vi "Motor Control (State Machine).vi"() -> ()   [LabVIEW 2013]
uses:
  <vilib>/eio/EIONode/EIONode.xnode
  <vilib>/rvi/eio/common/nirviEmuTemplateMethod_errors.vi
panel:
  in  "stop":bool
  in  "Update":bool
  out "Inside values":T1
  in  "Control":T1={"Pulse Lenght DIO3"=10000, "Pulse Period 3"=20000, "Angle"=0}
  in  "Position Reset":bool
  out "Position (Counts)":i64
  in  "Velocity Interval (uSec)":u64
  out "Acceleration (Counts/Interval)":i64
  out "Velocity (Counts/Interval)":i64
  out "Tours":i64
  out "Degree (relative)":i64
  out "Degree (absolute)":i64
  out "Pulses":i64
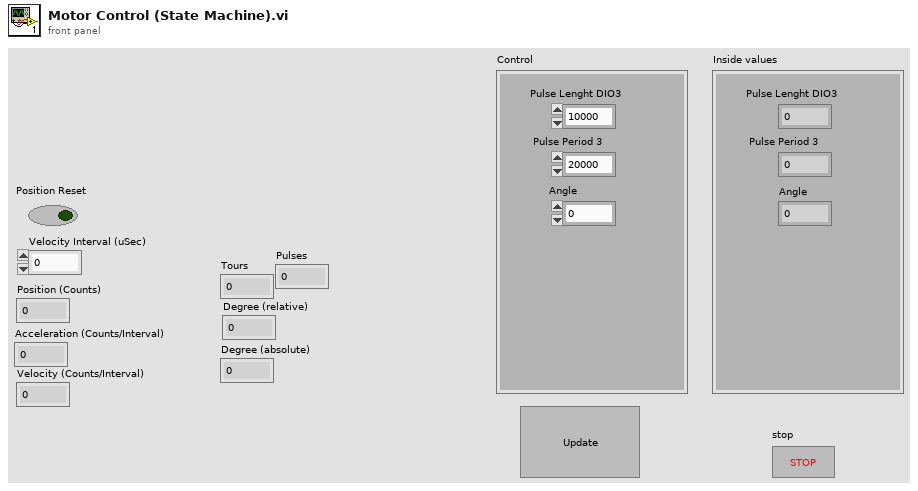
[diagram p1: front panel]
types:
  T1 = cluster{"Pulse Lenght DIO3":i16, "Pulse Period 3":i16, "Angle":i16}
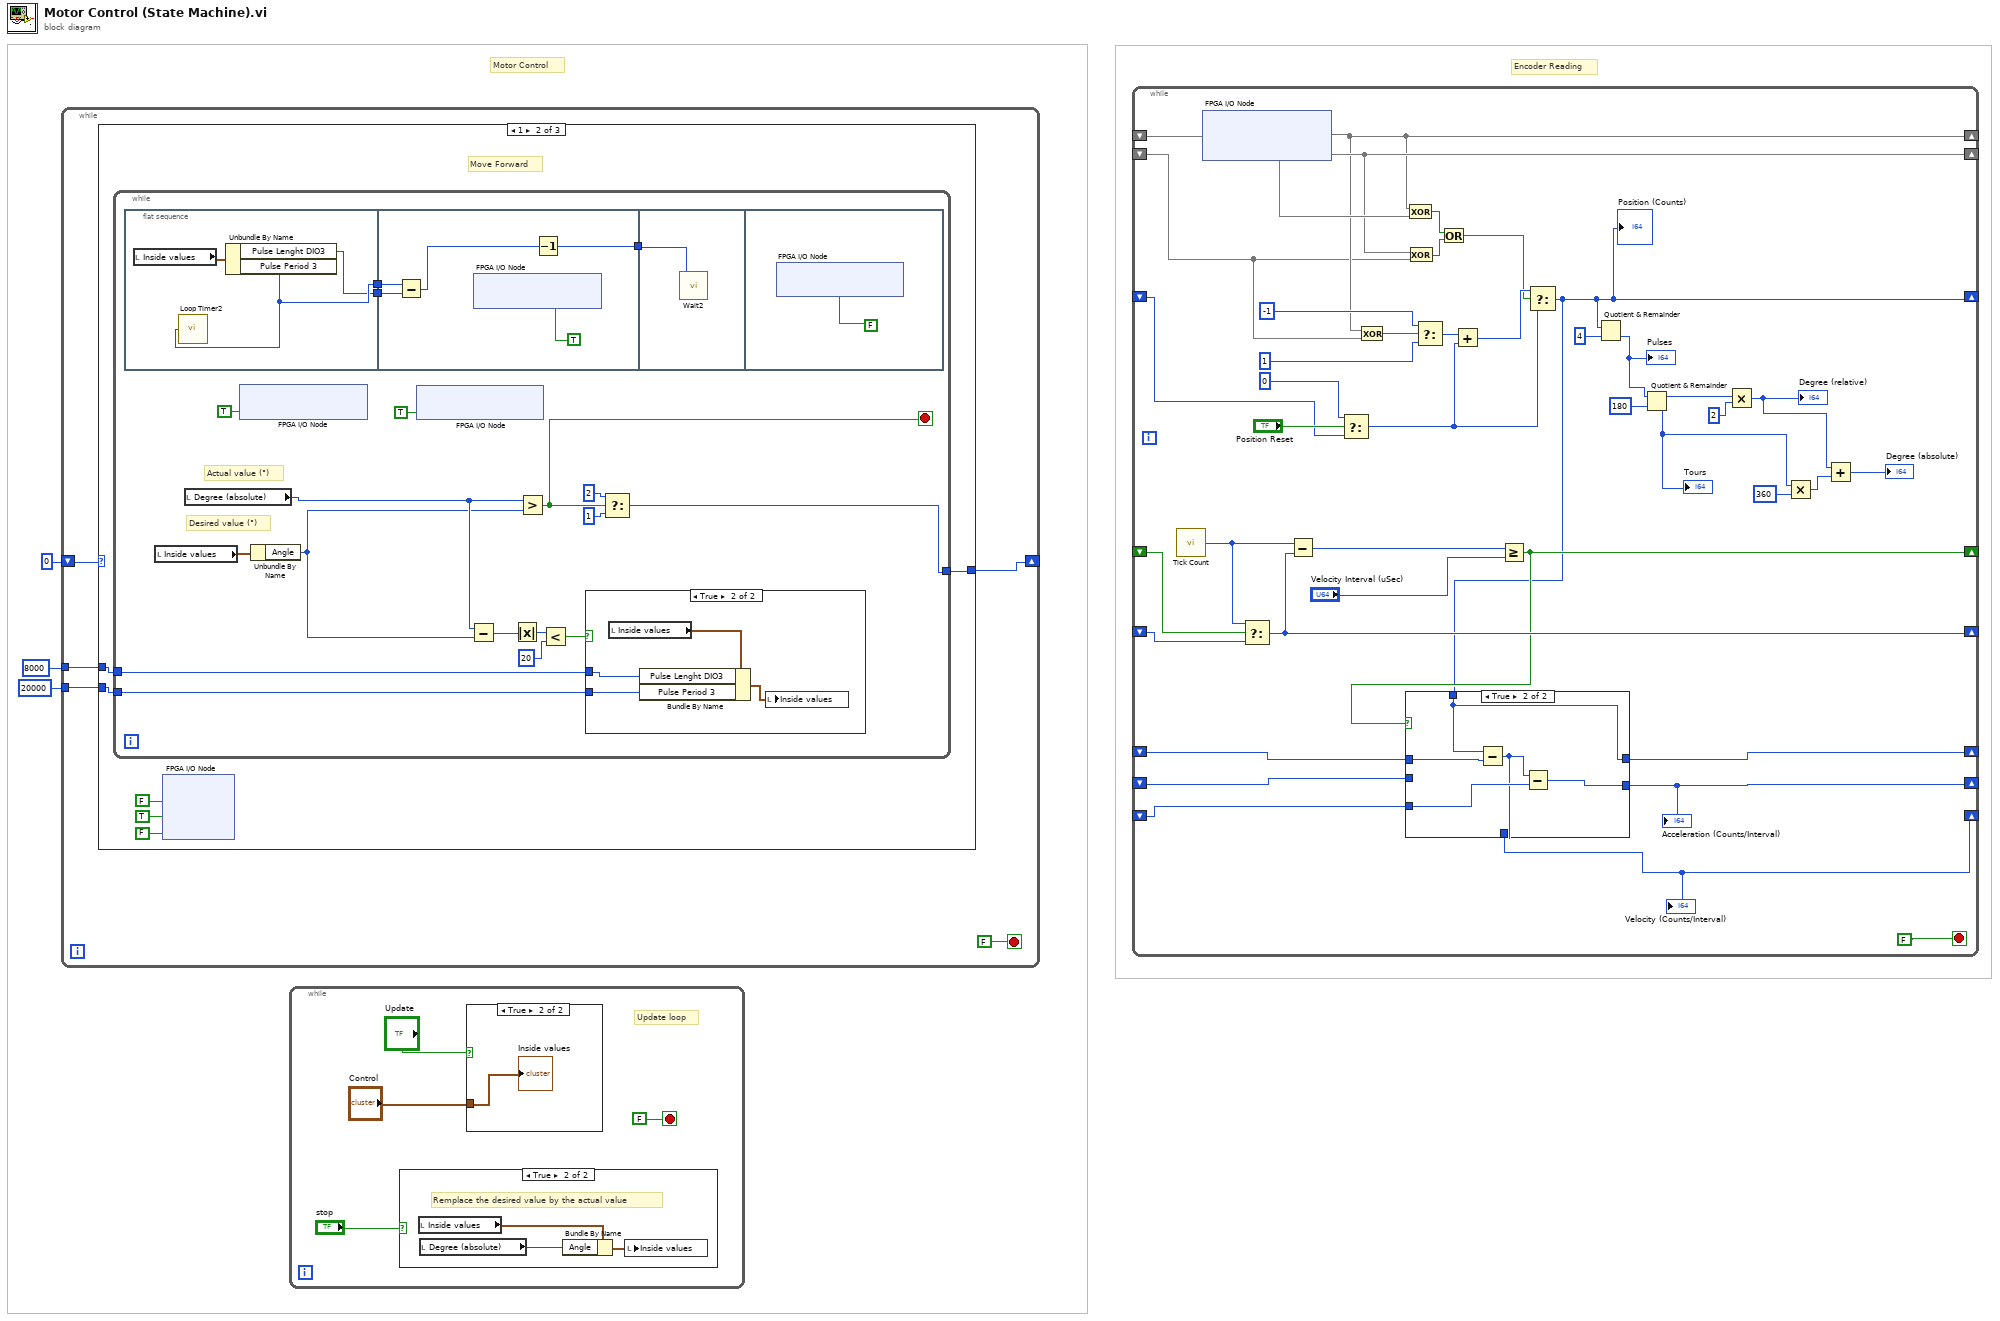
[diagram p0: block diagram]
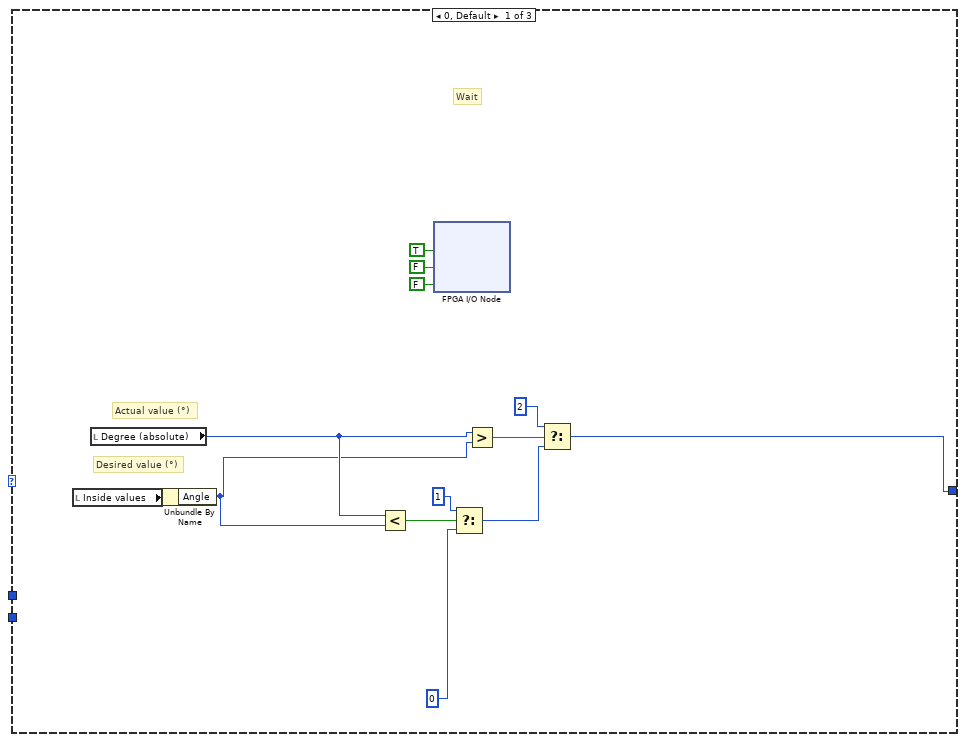
[diagram p5: hidden frame]
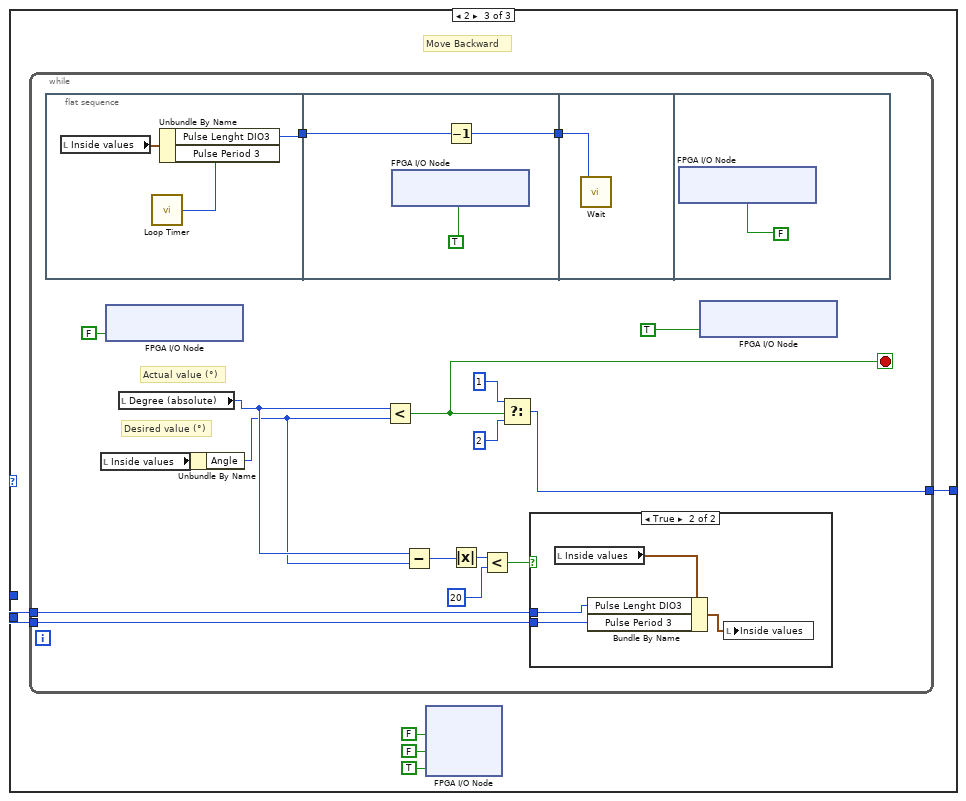
[diagram p7: hidden frame]
diagram:
  # "Motor Control"
  # "Encoder Reading"
  n1 = while {
    shift-right: [w7] -> _
    shift-left: i16 0 -> [w8]
    tunnel: i16 8000 -> [w5]
    tunnel: i16 20000 -> [w4]
    stop <- FALSE stop-if-true
    n2 = case shown="1" w8 {
      tunnel: [w15 w24 w62] -> w7
      tunnel: w5 -> [_ w23 w61]
      tunnel: w4 -> [_ w22 w60]
      frame 0, Default {
        # "Desired value (°)"
        # "Actual value (°)"
        # "Wait"
        n3 = local read "Inside values"() -> (w11:T1)
        n4 = local read "Degree (absolute)"() -> (w10:i64)
        n5 = Unbundle By Name(w11) -> ("Angle"=w9:i16)
        n6 = Less?(x=w10, y=w9) -> (x < y?=w20:bool)
        n7 = xnode "FPGA I/O Node"("LED0"=TRUE, "LED1"=FALSE, "LED2"=FALSE) -> ()  [unwired: 3 in, 3 out]
        n8 = Select(t=i16 1, s=w20, f=i16 0) -> (s? t:f=w17:i16)
        n9 = Greater?(x=w10, y=w9) -> (0:w21:bool)
        n10 = Select(t=i16 2, s=w21, f=w17) -> (s? t:f=w15:i16)
      }
      frame 1 {
        # "Move Forward"
        n11 = while {
          tunnel: [w37] -> w24
          tunnel: w22 -> [w29]
          tunnel: w23 -> [w28]
          stop <- w36 stop-if-true
          # "Desired value (°)"
          # "Actual value (°)"
          n12 = flat-sequence {
            tunnel: [w52] -> w44
            tunnel: [w51] -> w43
            tunnel: [w56] -> w45
            tunnel: w44 -> [w55]
            tunnel: w43 -> [w54]
            tunnel: w45 -> [w58]
            frame #0 {
              n13 = local read "Inside values"() -> (w50:T1)
              n14 = Unbundle By Name(w50) -> ("Pulse Lenght DIO3"=w51:i16, "Pulse Period 3"=w52:i16)
              n15 = call "Loop Timer2"("Count(Ticks)"=w52) -> ()  [unwired: 1 out]
            }
            frame #1 {
              n16 = Subtract(x=w55, y=w54) -> (x-y=w53:i16)
              n17 = xnode "FPGA I/O Node"("ConnectorB/DIO1"=TRUE ("ConnectorC/DIO7")) -> ()  [unwired: 1 in, 1 out]
              n18 = Decrement(x=w53) -> (x-1=w56:i16)
            }
            frame #2 {
              n19 = call "Wait2"("Count(Ticks)"=w58) -> ()  [unwired: 1 out]
            }
            frame #3 {
              n20 = xnode "FPGA I/O Node"("ConnectorB/DIO1"=FALSE ("ConnectorC/DIO7")) -> ()  [unwired: 1 in, 1 out]
            }
          }
          n21 = local read "Inside values"() -> (w40:T1)
          n22 = local read "Degree (absolute)"() -> (w31:i64)
          n23 = xnode "FPGA I/O Node"("ConnectorB/DIO2"=TRUE ("ConnectorC/DIO7")) -> ()  [unwired: 1 in, 1 out]
          n24 = Unbundle By Name(w40) -> ("Angle"=w30:i16)
          n25 = xnode "FPGA I/O Node"("ConnectorB/DIO0"=TRUE ("ConnectorA/DIO0")) -> ()  [unwired: 1 in, 1 out]
          n26 = Subtract(x=w31, y=w30) -> (x-y=w32:i64)
          n27 = Absolute Value(x=w32) -> (abs(x)=w33:i64)
          n28 = Greater?(x=w31, y=w30) -> (0:w36:bool)
          n29 = Less?(x=w33, y=i16 20) -> (x < y?=w34:bool)
          n30 = case shown="True" w34 {
            tunnel: w29 -> [_ w47]
            tunnel: w28 -> [_ w46]
            frame False {
            }
            frame True {
              n31 = local read "Inside values"() -> (w49:T1)
              n32 = Bundle By Name(cluster=w49, "Pulse Lenght DIO3"=w46, "Pulse Period 3"=w47) -> (w48:T1)
              n33 = local write "Inside values"(w48) -> ()
            }
          }
          n34 = Select(t=i16 2, s=w36, f=i16 1) -> (s? t:f=w37:i16)
        }
        n35 = xnode "FPGA I/O Node"("LED0"=FALSE, "LED1"=TRUE, "LED2"=FALSE) -> ()  [unwired: 3 in, 3 out]
      }
      frame 2 {
        # "Move Backward"
        n36 = while {
          tunnel: [w76] -> w62
          tunnel: w61 -> [w67]
          tunnel: w60 -> [w66]
          stop <- w74 stop-if-true
          # "Desired value (°)"
          # "Actual value (°)"
          n37 = flat-sequence {
            tunnel: [w88] -> w82
            tunnel: w82 -> [w90]
            tunnel: [w91] -> w81
            tunnel: w81 -> [w93]
            frame #0 {
              n38 = local read "Inside values"() -> (w87:T1)
              n39 = Unbundle By Name(w87) -> ("Pulse Lenght DIO3"=w88:i16, "Pulse Period 3"=w89:i16)
              n40 = call "Loop Timer"("Count(Ticks)"=w89) -> ()  [unwired: 1 out]
            }
            frame #1 {
              n41 = xnode "FPGA I/O Node"("ConnectorB/DIO1"=TRUE ("ConnectorC/DIO7")) -> ()  [unwired: 1 in, 1 out]
              n42 = Decrement(x=w90) -> (x-1=w91:i16)
            }
            frame #2 {
              n43 = call "Wait"("Count(Ticks)"=w93) -> ()  [unwired: 1 out]
            }
            frame #3 {
              n44 = xnode "FPGA I/O Node"("ConnectorB/DIO1"=FALSE ("ConnectorC/DIO7")) -> ()  [unwired: 1 in, 1 out]
            }
          }
          n45 = local read "Inside values"() -> (w75:T1)
          n46 = xnode "FPGA I/O Node"("ConnectorB/DIO2"=FALSE ("ConnectorC/DIO7")) -> ()  [unwired: 1 in, 1 out]
          n47 = local read "Degree (absolute)"() -> (w69:i64)
          n48 = Unbundle By Name(w75) -> ("Angle"=w68:i16)
          n49 = Less?(x=w69, y=w68) -> (x < y?=w74:bool)
          n50 = Subtract(x=w69, y=w68) -> (x-y=w70:i64)
          n51 = Absolute Value(x=w70) -> (abs(x)=w71:i64)
          n52 = Less?(x=w71, y=i16 20) -> (x < y?=w72:bool)
          n53 = Select(t=i16 1, s=w74, f=i16 2) -> (s? t:f=w76:i16)
          n54 = case shown="True" w72 {
            tunnel: w67 -> [_ w84]
            tunnel: w66 -> [_ w83]
            frame False {
            }
            frame True {
              n55 = local read "Inside values"() -> (w86:T1)
              n56 = Bundle By Name(cluster=w86, "Pulse Lenght DIO3"=w84, "Pulse Period 3"=w83) -> (w85:T1)
              n57 = local write "Inside values"(w85) -> ()
            }
          }
          n58 = xnode "FPGA I/O Node"("ConnectorB/DIO0"=TRUE ("ConnectorA/DIO0")) -> ()  [unwired: 1 in, 1 out]
        }
        n59 = xnode "FPGA I/O Node"("LED0"=FALSE, "LED1"=FALSE, "LED2"=TRUE) -> ()  [unwired: 3 in, 3 out]
      }
    }
  }
  n60 = while {
    stop <- FALSE stop-if-true
    # "Update loop"
    n61 = case shown="True" "stop" {
      frame False {
      }
      frame True {
        # "Remplace the desired value by the actual value"
        n62 = local read "Inside values"() -> (w101:T1)
        n63 = local read "Degree (absolute)"() -> (w100:i64)
        n64 = Bundle By Name(cluster=w101, "Angle"=w100) -> (w99:T1)
        n65 = local write "Inside values"(w99) -> ()
      }
    }
    n66 = case shown="True" "Update" {
      tunnel: "Control" -> [_ w102]
      frame False {
      }
      frame True {
        "Inside values" <- w102
      }
    }
  }
  n67 = while {
    shift-right: [w107] -> _
    shift-left: _ -> [w143]
    shift-right: [w120] -> _
    shift-left: _ -> [w106]
    shift-right: [w103] -> _
    shift-left: _ -> [w116]
    shift-right: [w128] -> _
    shift-left: _ -> [w131]
    shift-right: [w129] -> _
    shift-left: _ -> [w130]
    shift-right: [w126] -> _
    shift-left: _ -> [w127]
    shift-right: [w125] -> _
    shift-left: _ -> [w122]
    shift-right: [w123] -> _
    shift-left: _ -> [w124]
    stop <- FALSE stop-if-true
    n68 = call "Tick Count"() -> ("Tick Count(Ticks)"=w133:u32)
    n69 = xnode "FPGA I/O Node"() -> ("ConnectorA/DIO6"=w107, "ConnectorA/DIO7"=w120)  [unwired: 2 in, 2 out]
    n70 = Select(t=w133, s=w131, f=w130) -> (s? t:f=w129:u32)
    n71 = Subtract(x=w133, y=w129) -> (x-y=w134:u32)
    n72 = Select(t=i16 0, s="Position Reset", f=w116) -> (s? t:f=w135:i16)
    n73 = Exclusive Or(1:w106, 2:w107) -> (0:w119:bool)
    n74 = Exclusive Or(1:w143, 2:w107) -> (0:w142:bool)
    n75 = Exclusive Or(1:w106, 2:w120) -> (0:w141:bool)
    n76 = Select(t=i16 -1, s=w119, f=i16 1) -> (s? t:f=w137:i16)
    n77 = Or(x=w142, y=w141) -> (x .or. y?=w117:bool)
    n78 = Add(x=w137, y=w135) -> (x+y=w136:i16)
    n79 = Greater Or Equal?(x=w134, y="Velocity Interval (uSec)") -> (x >= y?=w128:bool)
    n80 = Select(t=w136, s=w117, f=w135) -> (s? t:f=w103:i16)
    "Position (Counts)" <- w103
    n81 = case shown="True" w128 {
      tunnel: w127 -> [w146 w151]
      tunnel: w103 -> [_ w150]
      tunnel: [w146 w150] -> w126
      tunnel: [w145 w149] -> w125
      tunnel: w124 -> [w144 w148]
      tunnel: [w144 w147] -> w123
      tunnel: w122 -> [w145 _]
      frame False {
      }
      frame True {
        n82 = Subtract(x=w150, y=w151) -> (x-y=w147:i16)
        n83 = Subtract(x=w147, y=w148) -> (x-y=w149:i16)
      }
    }
    "Acceleration (Counts/Interval)" <- w125
    "Velocity (Counts/Interval)" <- w123
    n84 = Quotient & Remainder(x=w103, y=i16 4) -> (floor(x/y)=w104:i16)  [unwired: 1 out]
    "Pulses" <- w104
    n85 = Quotient & Remainder(x=w104, y=i16 180) -> (x-y*floor(x/y)=w114:i16, floor(x/y)=w108:i16)
    "Tours" <- w108
    n86 = Multiply(x=w114, y=i16 2) -> (x*y=w111:i16)
    "Degree (relative)" <- w111
    n87 = Multiply(x=w108, y=i16 360) -> (x*y=w110:i16)
    n88 = Add(x=w111, y=w110) -> (x+y=→"Degree (absolute)":i16)
  }
